vi "IniGyro.vi"(10 "Gain (VoltsPerDegree/Second)":dbl=0.0125, 11 "refnum name":string="My Gyro RefNum") -> ()   [LabVIEW 2019]
uses:
  <vilib>/Rock Robotics/SystemInterfaces/spilib/spi_bus.ctl
  <vilib>/Rock Robotics/WPI/Gyro/WPI_GyroAnalogOpen.vi
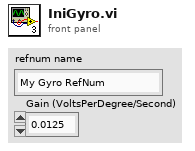
[diagram p1: front panel]
types:
  T1 = typedef "spi_bus.ctl" = enum16{"SPI On-Board, CS0", "SPI On-Board, CS1", "SPI On-Board, CS2", "SPI On-Board, CS3", "SPI MXP", "Invalid"}
  T2 = typedef "WPI_GyroDevRef.ctl" = cluster{"DevStatus":errorcluster, "Analog Channel":T3, "Gain (VoltsPerDegree/Second)":dbl, "Gyro Type":enum16{"Analog", "XRS450"}, "Handle":i32, "SPI Bus":T1, "Device Found":bool, "Sample Rate":dbl, "Calibrate On Open":bool, "Offset":dbl}
  T3 = typedef "FPGA_AIChannel.ctl" = enum8{"AI 0", "AI 1", "AI 2", "AI 3", "AI MXP 0", "AI MXP 1", "AI MXP 2", "AI MXP 3", "Invalid"}
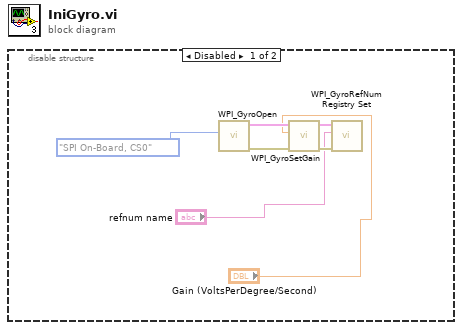
[diagram p0: block diagram]
diagram:
  n1 = disable-structure shown="Disabled" {
    frame Disabled {
      n2 = call-poly <vilib>:"WPI_GyroOpen.vi"("Analog Channel"=spi_bus."SPI On-Board, CS0" ("SPI Bus")) -> ("error out"=w4:errorcluster, "GyroDevRef"=w5:T2)  [unwired: 8 in, 1 out]
      n3 = call <vilib>:"WPI_GyroSetGain.vi"("error in (no error)"=w4, "Gain (VoltsPerDegree/Second)"="Gain (VoltsPerDegree/Second)", "GyroDevRef"=w5) -> ("error out"=w7:errorcluster, "GyroDevRef"=w6:T2)  [unwired: 7 in]
      n4 = call <vilib>:"WPI_GyroRefNum Registry Set.vi"("error in (no error)"=w7, "refnum name"="refnum name", "GyroDevRef"=w6) -> ()  [unwired: 7 in, 2 out]
    }
    frame Enabled {
    }
  }
